vi "ScaledDomains_subvi.vi"(10 "numbinsY":dbl, 11 "numbinsX":dbl) -> (2 "YDomainScaled":dbl[][](array[numeric]), 3 "XDomainScaled":dbl[][](array[numeric]))   [LabVIEW 2019]
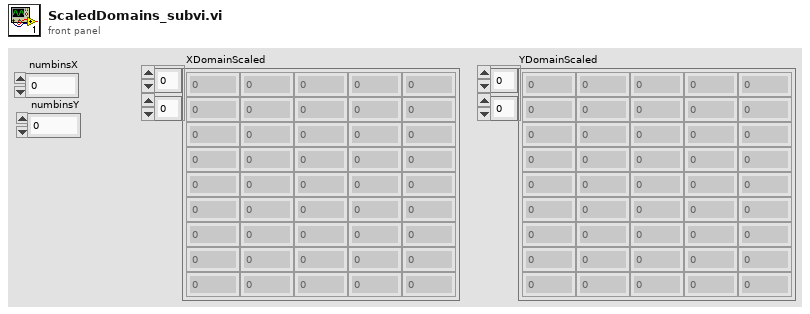
[diagram p1: front panel]
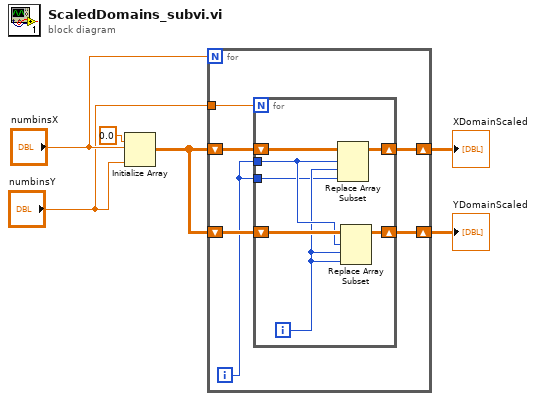
[diagram p0: block diagram]
diagram:
  n1 = Initialize Array(0.0 ("element"), "numbinsX", "numbinsY") -> (w5:dbl[][])
  n2 = for {
    N: "numbinsX" -> [_]
    shift-right: [w8] -> w2
    shift-left: w5 -> [w12]
    shift-right: [w7] -> w1
    shift-left: w5 -> [w11]
    tunnel: "numbinsY" -> [w9]
    i -> [w10]
    n3 = for {
      N: w9 -> [_]
      shift-right: [w14] -> w8
      shift-left: w12 -> [w19]
      shift-right: [w13] -> w7
      shift-left: w11 -> [w18]
      tunnel: w10 -> [w17]
      tunnel: w10 -> [w15]
      i -> [w16]
      n4 = Replace Array Subset(array=w19, new element=w15, index (row)=w17, index (col)=w16) -> (w14:dbl[][])
      n5 = Replace Array Subset(array=w18, new element=w16, index (row)=w17, index (col)=w16) -> (w13:dbl[][])
    }
  }
  "XDomainScaled" <- w2
  "YDomainScaled" <- w1
